vi "SpinnyCurrentPosMod.vi"(0 "Arduino Resource":T1={"VISA resource"="", "Board Type"=enum."Uno", "Connection Type"=enum."USB / Serial", "Bytes Per Packet (15)"=15}, 3 "stepper #":u8=1, 5 "error in":errorcluster) -> (14 "Arduino Resource Out":T1={"VISA resource"="", "Board Type"=enum."Uno", "Connection Type"=enum."USB / Serial", "Bytes Per Packet (15)"=15}, 18 "position":i32, 19 "error out":errorcluster)   [LabVIEW 2014]
doc: "return current position of nth stepper in steps"
uses:
  <vilib>/LabVIEW Interface for Arduino/Type Defs/Arduino Resource.ctl
  <vilib>/LabVIEW Interface for Arduino/Type Defs/Board Type.ctl
  <vilib>/LabVIEW Interface for Arduino/LabVIEW Interface for Arduino.lvlib
panel:
  out "Array":dbl[](array[numeric])
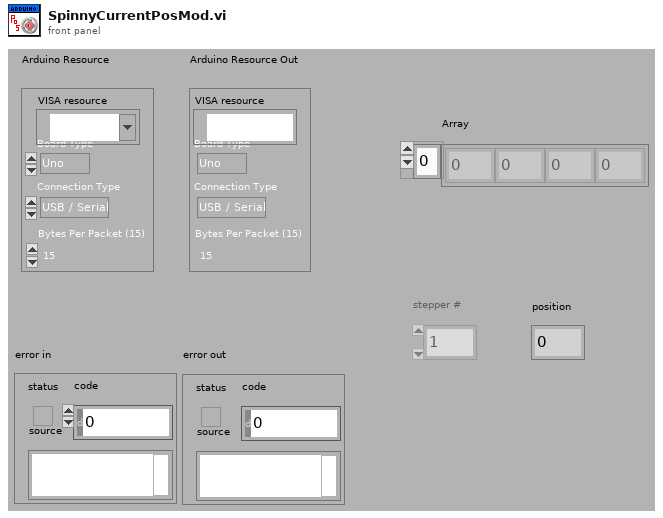
[diagram p1: front panel]
types:
  T1 = typedef "LabVIEW Interface for Arduino.lvlib/Arduino Resource.ctl" = cluster{"VISA resource":refnum<visa-resource-name>, "Board Type":T2, "Connection Type":enum8{"USB / Serial"}, "Bytes Per Packet (15)":u8}
  T2 = typedef "LabVIEW Interface for Arduino.lvlib/Board Type.ctl" = enum16{"Uno", "Dimuelanove w/Atmega 328", "Mega 2560"}
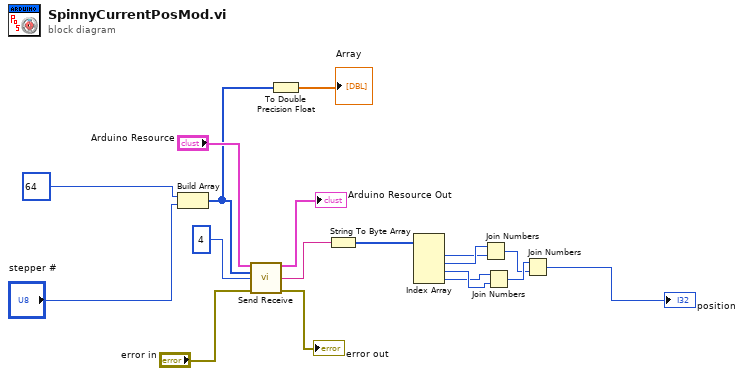
[diagram p0: block diagram]
diagram:
  n1 = Build Array(u8 64, "stepper #") -> (w2:u8[])
  n2 = call <vilib>:"Send Receive.vi"("Arduino Resource"="Arduino Resource", "Data"=w2, "Bytes To Read (0)"=u8 4, "error in"="error in") -> ("Arduino Resource"=→"Arduino Resource Out":T1, "Read Buffer"=w12:string, "error out"=→"error out":errorcluster)  [unwired: 9 in]
  n3 = To Double Precision Float(number=w2) -> (double precision float=→"Array":dbl[])
  n4 = String To Byte Array(string=w12) -> (unsigned byte array=w11:u8[])
  n5 = Index Array(array=w11) -> (element #1=w9:u8, element #2=w10:u8, element #3=w7:u8, element #4=w6:u8)  [unwired: 4 in]
  n6 = Join Numbers(hi=w10, lo=w9) -> ((hi.lo)=w4:u16)
  n7 = Join Numbers(hi=w6, lo=w7) -> ((hi.lo)=w5:u16)
  n8 = Join Numbers(hi=w5, lo=w4) -> ((hi.lo)=→"position":u32)
